vi "Write Beep Parameters.vi"(7 "Use System Alert?":bool, 8 "error in (no error)":errorcluster, 9 "Duration":dbl[unit]=0.1, 10 "Frequency (440)":dbl[unit]=440.0, 11 "Beep in":refnum<class "Beep.lvclass">) -> (0 "error out":errorcluster, 3 "Beep out":refnum<class "Beep.lvclass">)   [LabVIEW 2016, in "CS++BeepActor.lvlib" / "Beep.lvclass"]
doc: "Set some parameters for beep generation."
uses:
  Beep.lvclass
  Beep.lvclass/Beep.ctl
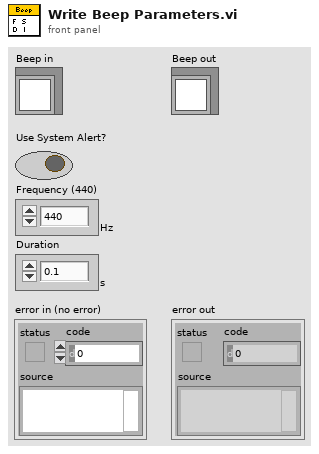
[diagram p1: front panel]
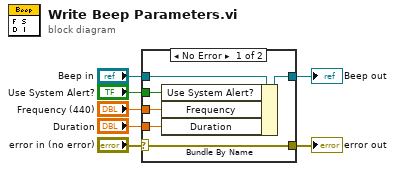
[diagram p0: block diagram]
diagram:
  n1 = case shown="No Error" "error in (no error)" {
    selector: "error in (no error)" -> [w13 w15]
    tunnel: [w13 w15] -> w6
    tunnel: [w11 w14] -> w4
    tunnel: "Beep in" -> [w12 w14]
    tunnel: "Use System Alert?" -> [w10 _]
    tunnel: "Frequency (440)" -> [w9 _]
    tunnel: "Duration" -> [w8 _]
    frame No Error {
      n2 = Bundle By Name(cluster=w12, "Use System Alert?"=w10, "Frequency"=w9, "Duration"=w8) -> (w11:refnum<class "Beep.lvclass">)
    }
    frame Error {
    }
  }
  "error out" <- w6
  "Beep out" <- w4
